vi "Filter Wheel Test.vi"(8 "error in (no error)":errorcluster, 11 "Session Handle in":T1) -> (0 "error out":errorcluster, 2 "Passed?":bool, 3 "Session Handle out":T1 caption="Gas")   [LabVIEW 2015, in "PAS.lvclass"]
uses:
  PAS.lvclass
  Typedefs/Session Handle.ctl
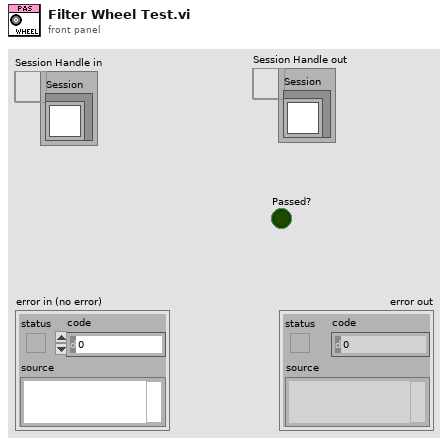
[diagram p1: front panel]
types:
  T1 = typedef "PAS.lvclass/Session Handle.ctl" = refnum<data-value>
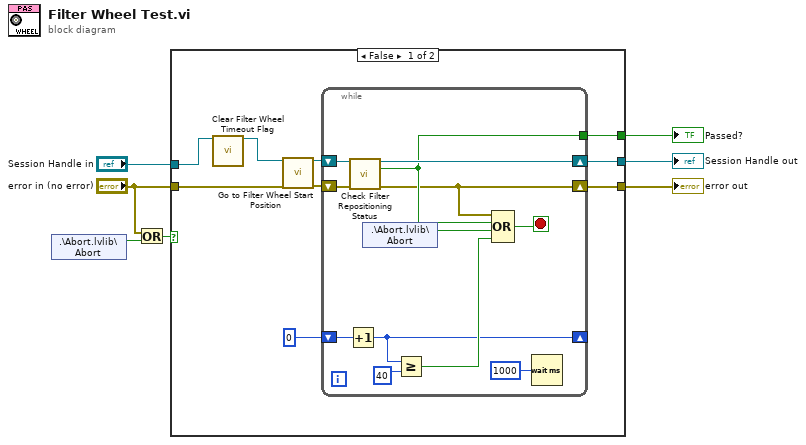
[diagram p0: block diagram]
diagram:
  n1 = shared-variable ".\\Abort.lvlib\\Abort"() -> (w1:bool)  [unwired: 1 in, 1 out]
  n2 = Or(x="error in (no error)", y=w1) -> (x .or. y?=w3:bool)
  n3 = case shown="False" w3 {
    tunnel: [w16 w29] -> w7
    tunnel: [w15 _] -> w6
    tunnel: [w11 w30] -> w5
    tunnel: "Session Handle in" -> [w10 w30]
    tunnel: "error in (no error)" -> [w8 w29]
    frame False {
      n4 = call "Clear Filter Wheel Timeout Flag.vi"("Session Handle in"=w10) -> ("Session Handle out"=w9:T1)  [unwired: 11 in, 3 out]
      n5 = call "Go to Filter Wheel Start Position.vi"("Session Handle in"=w9, "error in (no error)"=w8) -> ("Session Handle out"=w13:T1, "error out"=w12:errorcluster)  [unwired: 12 in]
      n6 = while {
        shift-right: [w18] -> w16
        shift-left: w12 -> [w22]
        shift-right: [w20] -> w11
        shift-left: w13 -> [w21]
        tunnel: [w19] -> w15
        shift-right: [w23] -> _
        shift-left: u32 0 ("milliseconds to wait") -> [w26]
        stop <- w27 stop-if-true
        n7 = Increment(x=w26) -> (x+1=w23:u32)
        n8 = call "Check Filter Repositioning Status.vi"("Session Handle in"=w21, "error in (no error)"=w22) -> ("Session Handle out"=w20:T1, "Success?"=w19:bool, "error out"=w18:errorcluster)  [unwired: 11 in]
        n9 = shared-variable ".\\Abort.lvlib\\Abort"() -> (w17:bool)  [unwired: 1 in, 1 out]
        n10 = Greater Or Equal?(x=w23, y=u32 40) -> (x >= y?=w24:bool)
        n11 = Compound Arithmetic op=OR(w18, w19, w17, w24) -> (w27:bool)
        n12 = Wait (ms)(milliseconds to wait=u32 1000) -> ()  [unwired: 1 out]
      }
    }
    frame True {
    }
  }
  "error out" <- w7
  "Passed?" <- w6
  "Session Handle out" <- w5
